vi "LinkNodes.vi"(8 "error in (no error)":errorcluster, 9 "GraphNode2 in":refnum<data-value>, 10 "GraphNode1 in":refnum<data-value>) -> (0 "error out":errorcluster, 1 "GraphNode2 out":refnum<data-value>, 2 "GraphNode1 out":refnum<data-value>)   [LabVIEW 2009, in "Graph.lvclass"]
doc: "Links two graph nodes together."
uses:
  Graph.lvclass
  GraphNode/GraphNode.lvclass
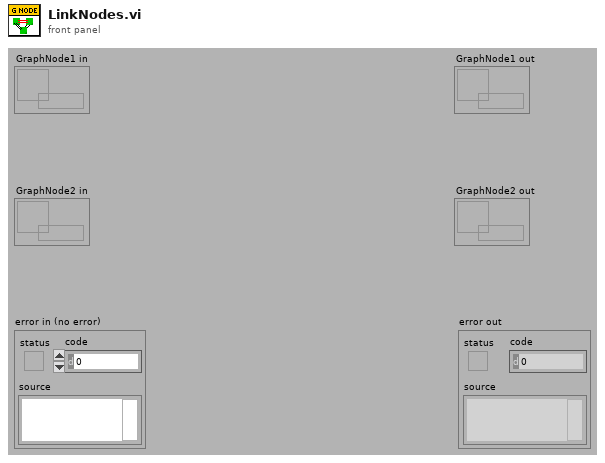
[diagram p1: front panel]
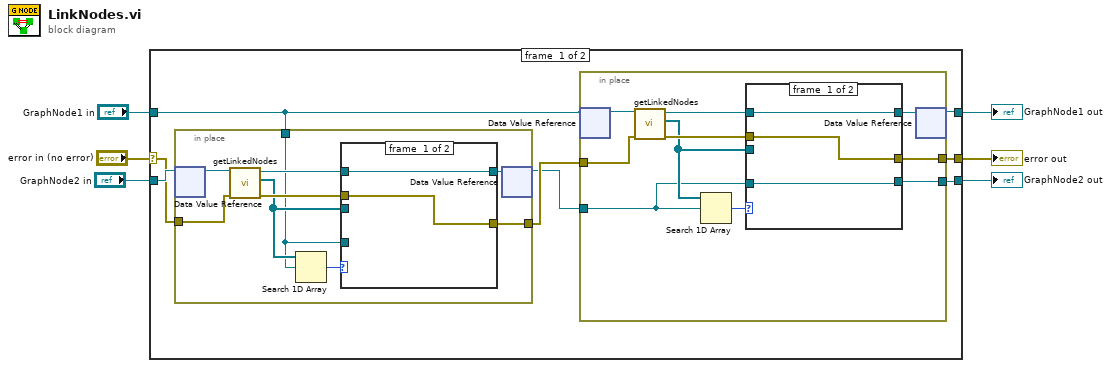
[diagram p0: block diagram]
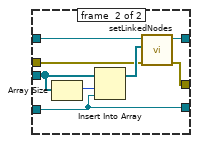
[diagram p2: hidden frame]
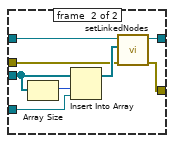
[diagram p3: hidden frame]
diagram:
  n1 = case shown="No Error" "error in (no error)" {
    selector: "error in (no error)" -> [w13 w57]
    tunnel: [w7 w57] -> w5
    tunnel: "GraphNode1 in" -> [w11 w55]
    tunnel: "GraphNode2 in" -> [w14 w56]
    tunnel: [w12 w55] -> w2
    tunnel: [w8 w56] -> w1
    frame #0 {
      n2 = in-place {
        in-place-border: w13 -> [w43]
        in-place-border: w11 -> [w36]
        in-place-border: [w40] -> w10
        n3 = in-place-dvr #1(w14) -> (w44:refnum<class "GraphNode.lvclass">)  [unwired: 1 out]
        n4 = call "getLinkedNodes.vi"("error in (no error)"=w43, "GraphNode in"=w44) -> ("error out"=w41:errorcluster, "LinkedNodes"=w38:refnum<data-value>[], "GraphNode out"=w42:refnum<class "GraphNode.lvclass">)  [unwired: 7 in]
        n5 = Search 1D Array(1D array=w38, element=w36) -> (index of element=w37:i32)  [unwired: 1 in]
        n6 = case shown="-1" w37 {
          tunnel: w42 -> [w46 w54]
          tunnel: w41 -> [w45 w52]
          tunnel: [w45 w51] -> w40
          tunnel: [w46 w50] -> w39
          tunnel: w38 -> [_ w49]
          tunnel: w36 -> [_ w47]
          frame #0 {
          }
          frame #1 {
            n7 = Array Size(array=w49) -> (size(s)=w48:i32)
            n8 = Insert Into Array(array=w49, index=w48, new element=w47) -> (w53:refnum<data-value>[])
            n9 = call "setLinkedNodes.vi"("error in (no error)"=w52, "LinkedNodes"=w53, "GraphNode in"=w54) -> ("error out"=w51:errorcluster, "GraphNode out"=w50:refnum<class "GraphNode.lvclass">)  [unwired: 7 in]
          }
        }
        n10 = in-place-dvr #1(w39) -> (w9:refnum<data-value>)  [unwired: 1 out]
      }
      n11 = in-place {
        in-place-border: w10 -> [w23]
        in-place-border: w9 -> [w16]
        in-place-border: [w20] -> w7
        in-place-border: [w15] -> w8
        n12 = in-place-dvr #2(w11) -> (w24:refnum<class "GraphNode.lvclass">)  [unwired: 1 out]
        n13 = call "getLinkedNodes.vi"("error in (no error)"=w23, "GraphNode in"=w24) -> ("error out"=w21:errorcluster, "LinkedNodes"=w18:refnum<data-value>[], "GraphNode out"=w22:refnum<class "GraphNode.lvclass">)  [unwired: 7 in]
        n14 = Search 1D Array(1D array=w18, element=w16) -> (index of element=w17:i32)  [unwired: 1 in]
        n15 = case shown="-1" w17 {
          tunnel: w22 -> [w27 w35]
          tunnel: w21 -> [w26 w33]
          tunnel: [w26 w32] -> w20
          tunnel: [w27 w31] -> w19
          tunnel: w18 -> [_ w30]
          tunnel: w16 -> [w25 w28]
          tunnel: [w25 w28] -> w15
          frame #0 {
          }
          frame #1 {
            n16 = Array Size(array=w30) -> (size(s)=w29:i32)
            n17 = Insert Into Array(array=w30, index=w29, new element=w28) -> (w34:refnum<data-value>[])
            n18 = call "setLinkedNodes.vi"("error in (no error)"=w33, "LinkedNodes"=w34, "GraphNode in"=w35) -> ("error out"=w32:errorcluster, "GraphNode out"=w31:refnum<class "GraphNode.lvclass">)  [unwired: 7 in]
          }
        }
        n19 = in-place-dvr #2(w19) -> (w12:refnum<data-value>)  [unwired: 1 out]
      }
    }
    frame #1 {
    }
  }
  "error out" <- w5
  "GraphNode1 out" <- w2
  "GraphNode2 out" <- w1
